vi "SSS_V3.1.vi"() -> ()   [LabVIEW 2017]
uses:
  <vilib>/DAQmx/write.llb/DAQmx Write (Analog 2D DBL NChan NSamp).vi
  <vilib>/DAQmx/read.llb/DAQmx Read (Analog 1D Wfm NChan NSamp).vi
  <vilib>/DAQmx/create/channels.llb/DAQmx Create Channel (AO-Voltage-Basic).vi
  <vilib>/DAQmx/configure/timing.llb/DAQmx Timing (Sample Clock).vi
  <vilib>/DAQmx/miscellaneous.llb/DAQmx Fill In Error Info.vi
  <vilib>/DAQmx/create/channels.llb/DAQmx Create Channel (AI-Voltage-Basic).vi
panel:
  out "Sampling Rate(EN, OSC)":dbl format="%#_3p"
  in  "TXEN_Pulse length(sec)":dbl=0.0004 format="%#_6p"
  in  "OSC_Pulse length(sec)":dbl=0.0004 format="%#_6p"
  in  "GAIN_Pulse length(sec)":dbl=1.0 format="%#_6p"
  in  "STC_Sampling Frequency(Hz)":dbl=192000.0 format="%0.2f"
  in  "STC_STEP":enum16{"0", "1", "2", "3", "4", "5", "6", "7"}(ring)
  in  "STC_Pulse length(sec)":dbl=1.0 format="%#_6p"
  in  "OSC_Frequency(Hz)":dbl=430000.0 format="%#_6p"
  in  "디바이스 이름(DAQ4)":tag="Dev4"
  in  "송신채널(DAQ4)":tag="Dev4/ao0:1"
  in  "송신채널(DAQ5)":tag="Dev5/ao0:1"
  in  "디바이스 이름(DAQ5)":tag="Dev5"
  in  "송신채널(DAQ3)":tag="Dev3/ao0:1"
  in  "Samplig Rate(RX)":dbl=1500000.0
  in  "RX time(sec)":dbl=0.0004
  out "RX.CH2 2":waveform(dbl)(graph)
  out "RX.CH2":waveform(dbl)(graph)
  in  "Start Frequency(Hz)":dbl=430000.0 format="%#_6p"
  in  "Pulse length(sec)":dbl=4e-06 format="%#_6p"
  in  "sampling rate(TX)":dbl=3760000.0 caption="Sampling Rate(TX)" format="%#.2g"
  in  "STEP":i32=100
  in  "초기 위상":dbl format="%#_13g"
  in  "Bandwidth":dbl=40000.0 format="%#_6p"
  out "Hz/1STEP":dbl
  out "TX.CH1":waveform(dbl)(graph)
  out "TX Spectrum":cluster{"f0":dbl, "df":dbl, "magnitude":dbl[]}(graph)
  out "TX.CH 2":waveform(dbl)(graph)
  in  "디바이스 이름(DAQ3)":tag="Dev3"
  in  "수신채널(DAQ3)":tag="Dev3/ai0:1"
  in  "Number of Sample":i32=150000 format="%#.0g"
  out "불리언 2":bool
  in  "Signal_Processing 2":bool
  out "CMD_PWD_DATA":i32=4
  in  "Signal_Processing":bool
  out "CMD_PWD":i32=7
  out "CMD_TVG":i32=6
  out "CMD_TVG_DATA":i32=4
  out "CMD_GAIN":i32=5
  out "CMD_GAIN_DATA":i32=255
  out "CMD_RANGE":i32=4
  out "CMD_RANGE_DATA":i32=100
  out "CMD_STOP":i32=3
  out "CMD_STOP_DATA":i32
  out "CMD_START":i32=2
  out "CMD_START_DATA":i32=1
  in  "port":u16=2500
  in  "address":string="30.0.1.18"
  in  "TCP/IP":bool
  in  "Server Closed":string="The server VI closed the connection."
  # "TCP/IP 소켓 통신 설정"
  # "송신 신호 변조 설정"
  # "수신 신호 변조 설정"
  # "DAQ Max 설정"
  # "DAQ3"
  # "DAQ5"
  # "DAQ4"
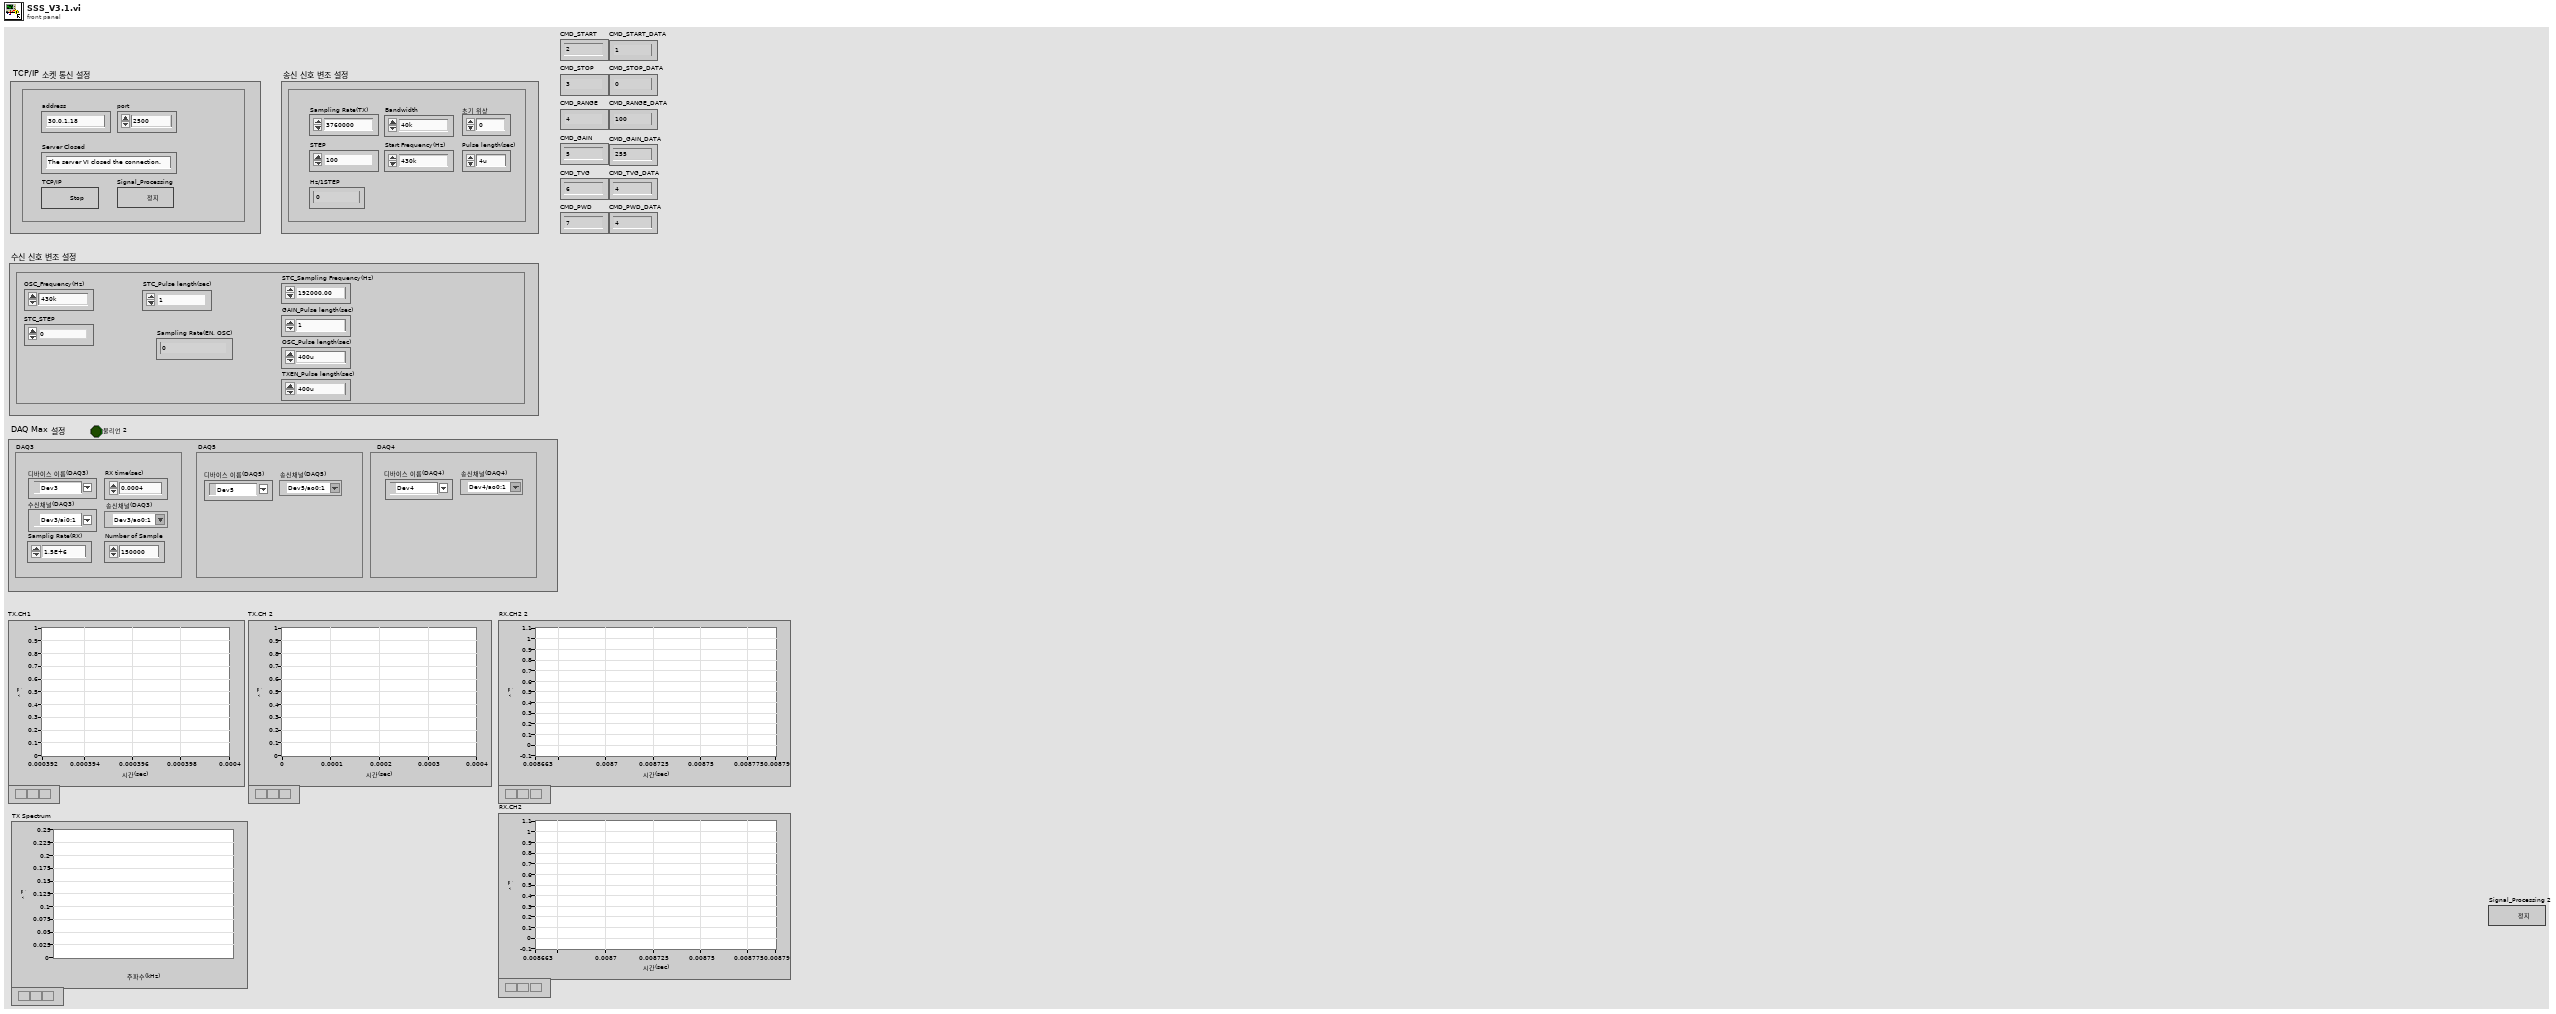
[diagram p1: front panel]
types:
  T1 = enum16{"Standard", "Buffered", "CRLF", "Immediate"}
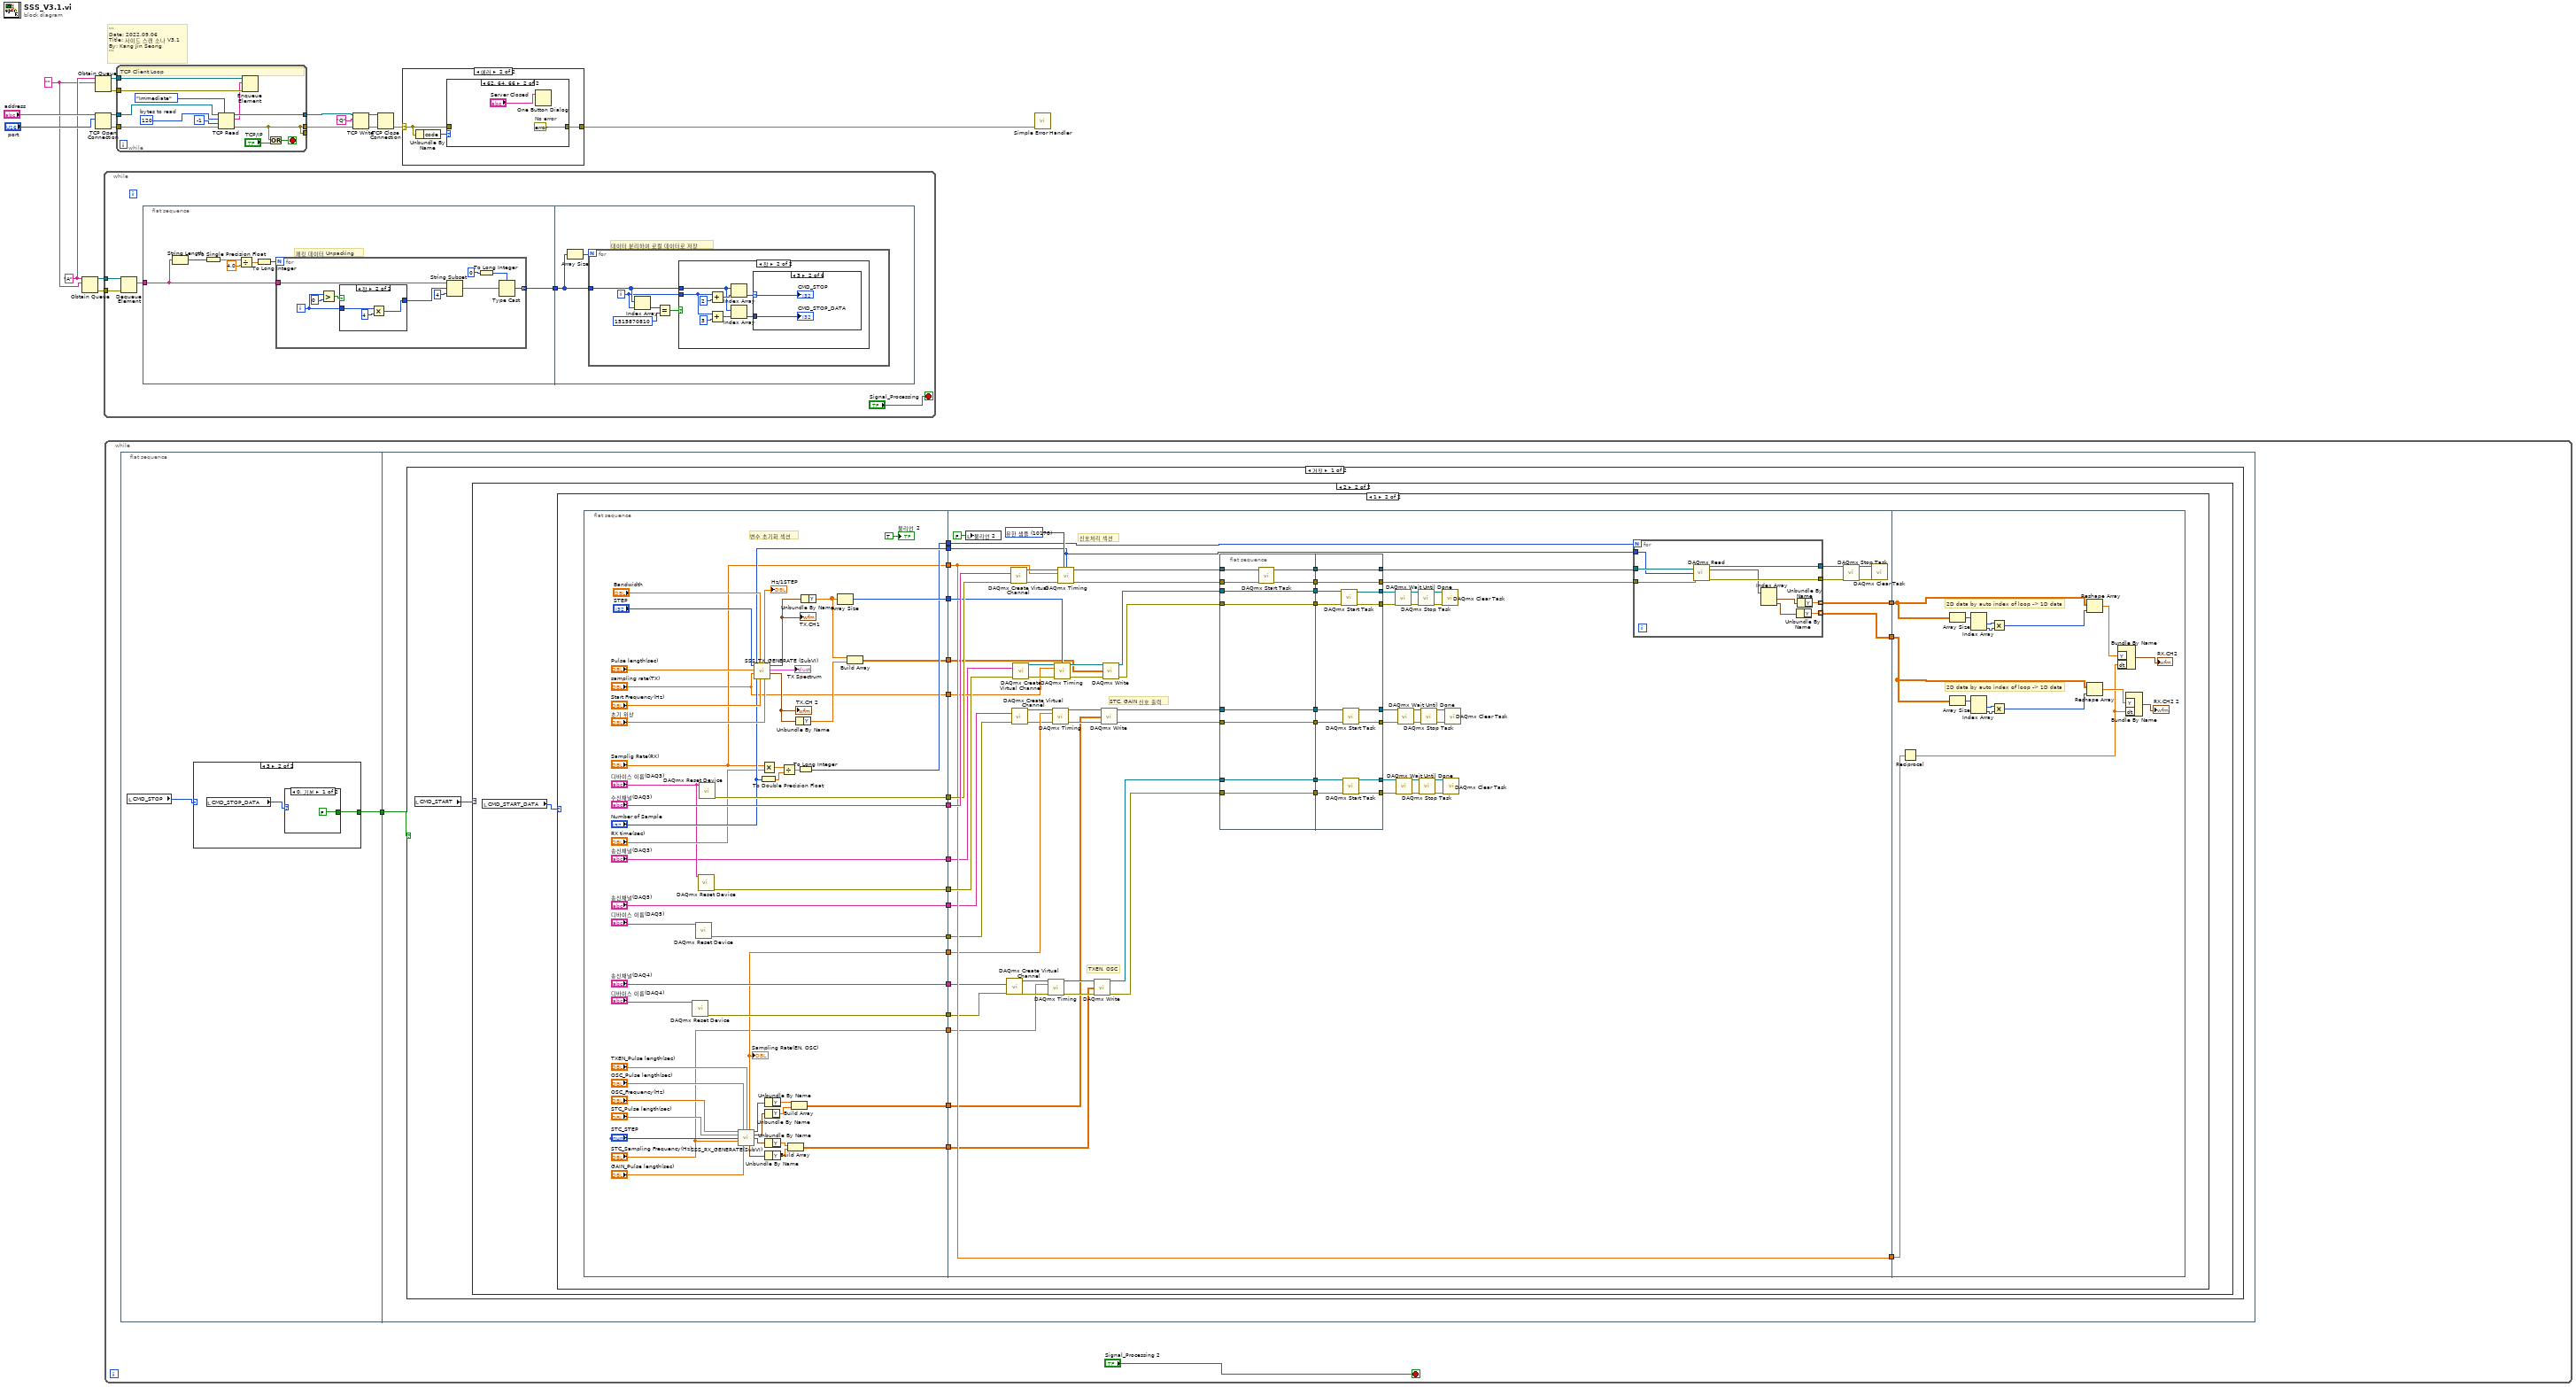
[diagram p0: block diagram]
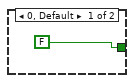
[diagram p2: hidden frame]
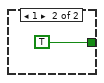
[diagram p3: hidden frame]
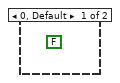
[diagram p4: hidden frame]
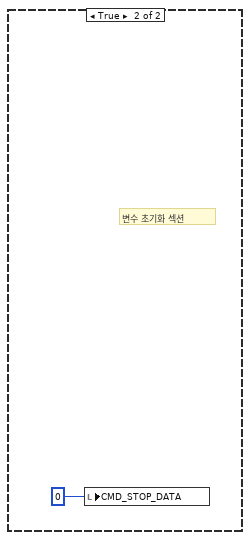
[diagram p6: hidden frame]
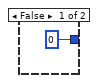
[diagram p7: hidden frame]
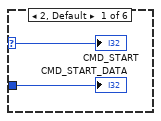
[diagram p9: hidden frame]
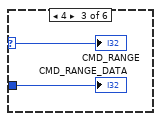
[diagram p10: hidden frame]
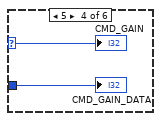
[diagram p11: hidden frame]
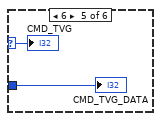
[diagram p12: hidden frame]
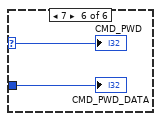
[diagram p13: hidden frame]
diagram:
  w1 = ""
  w4 = "A" ("이름(이름없음)")
  # "'''\nDate: 2022.09.06\nTitle: 사이드 스캔 소나 V3.1\nBy: Kang Jin Seong\n'''"
  n1 = Obtain Queue(name (unnamed)=w4, element data type=w1) -> (queue out=w3:refnum<queue>, error out=w2:errorcluster)  [unwired: 3 in, 1 out]
  n2 = Obtain Queue(name (unnamed)=w4, element data type=w1) -> (queue out=w6:refnum<queue>, error out=w5:errorcluster)  [unwired: 3 in, 1 out]
  n3 = TCP Open Connection(address="address", remote port or service name="port") -> (connection ID=w7:refnum<k5>, error out=w8:errorcluster)  [unwired: 3 in]
  n4 = while {
    tunnel: w3 -> [w21]
    tunnel: w2 -> [w20]
    stop <- "Signal_Processing" stop-if-true
    n5 = Dequeue Element(queue=w21, error in (no error)=w20) -> (element=w19:string)  [unwired: 1 in, 3 out]
    n6 = flat-sequence {
      tunnel: w19 -> [w25]
      tunnel: [w23] -> w22
      tunnel: w22 -> [w44]
      frame #0 {
        # "패킷 데이터 Unpacking"
        n7 = String Length(string=w25) -> (length=w29:i32)
        n8 = To Single Precision Float(number=w29) -> (single precision float=w28:sgl)
        n9 = Divide(x=w28, y=sgl 4.0) -> (x/y=w26:sgl)
        n10 = To Long Integer(number=w26) -> (32bit integer=w24:i32)
        n11 = for {
          N: w24 -> [_]
          tunnel: w25 -> [w39]
          tunnel: [w36] -> w23 mode=indexing
          i -> [w31]
          n12 = Greater?(x=w31, y=0) -> (0:w33:bool)
          n13 = case shown="참" w33 {
            tunnel: [0 w41] -> w32
            tunnel: w31 -> [_ w43]
            frame False {
            }
            frame True {
              n14 = Multiply(x=w43, y=4) -> (x*y=w41:i32)
            }
          }
          n15 = String Subset(string=w39, offset (0)=w32, length (rest)=4 ("길이(나머지)")) -> (substring=w30:string)
          n16 = To Long Integer(number=0 ("숫자")) -> (32bit integer=w38:i32)
          n17 = Type Cast(type=w38, x=w30) -> (*(type *) &x=w36:i32)
        }
      }
      frame #1 {
        # "데이터 분리하여 로컬 데이터로 저장"
        n18 = Array Size(array=w44) -> (size(s)=w45:i32)
        n19 = for {
          N: w45 -> [_]
          tunnel: w44 -> [w47]
          i -> [w46]
          n20 = Index Array(array=w47, index=w46) -> (element=w50:i32)
          n21 = Equal?(x=w50, y=1515870810) -> (x = y?=w48:bool)
          n22 = case shown="참" w48 {
            tunnel: w47 -> [_ w52]
            tunnel: w46 -> [_ w53]
            frame False {
            }
            frame True {
              n23 = Add(x=w53, y=2) -> (x+y=w57:i32)
              n24 = Add(x=w53, y=3) -> (x+y=w54:i32)
              n25 = Index Array(array=w52, index=w57) -> (element=w56:i32)
              n26 = Index Array(array=w52, index=w54) -> (element=w51:i32)
              n27 = case shown="3" w56 {
                selector: w56 -> [w60 w62 w64 w66 w68 w70]
                tunnel: w51 -> [w59 w61 w63 w65 w67 w69]
                frame 2, Default {
                  "CMD_START" <- w60
                  "CMD_START_DATA" <- w59
                }
                frame 3 {
                  "CMD_STOP" <- w62
                  "CMD_STOP_DATA" <- w61
                }
                frame 4 {
                  "CMD_RANGE" <- w64
                  "CMD_RANGE_DATA" <- w63
                }
                frame 5 {
                  "CMD_GAIN" <- w66
                  "CMD_GAIN_DATA" <- w65
                }
                frame 6 {
                  "CMD_TVG" <- w68
                  "CMD_TVG_DATA" <- w67
                }
                frame 7 {
                  "CMD_PWD" <- w70
                  "CMD_PWD_DATA" <- w69
                }
              }
            }
          }
        }
      }
    }
  }
  n28 = while {
    stop <- "Signal_Processing 2" stop-if-true
    n29 = flat-sequence {
      tunnel: [w73] -> w71
      tunnel: w71 -> [w80]
      frame #0 {
        n30 = local read "CMD_STOP"() -> (w74:i32)
        n31 = case shown="3" w74 {
          tunnel: [FALSE w76] -> w73
          frame 0, Default {
          }
          frame 3 {
            n32 = local read "CMD_STOP_DATA"() -> (w77:i32)
            n33 = case shown="0, 기본" w77 {
              tunnel: [FALSE TRUE] -> w76
              frame 0, Default {
              }
              frame 1 {
              }
            }
          }
        }
      }
      frame #1 {
        n34 = case shown="거짓" w80 {
          frame False {
            n35 = local read "CMD_START"() -> (w81:i32)
            n36 = case shown="2" w81 {
              frame 0, Default {
                (unwired) FALSE
              }
              frame 2 {
                n37 = local read "CMD_START_DATA"() -> (w82:i32)
                n38 = case shown="1" w82 {
                  frame 0, Default {
                  }
                  frame 1 {
                    n39 = flat-sequence {
                      tunnel: ["수신채널(DAQ3)"] -> w103
                      tunnel: [w142] -> w102
                      tunnel: ["Samplig Rate(RX)"] -> w101
                      tunnel: ["Number of Sample"] -> w100
                      tunnel: [w140] -> w99
                      tunnel: [w138] -> w98
                      tunnel: [w137] -> w97
                      tunnel: [w133] -> w93
                      tunnel: ["송신채널(DAQ3)"] -> w92
                      tunnel: [w128] -> w91
                      tunnel: ["송신채널(DAQ5)"] -> w90
                      tunnel: ["sampling rate(TX)"] -> w89
                      tunnel: [w110] -> w88
                      tunnel: ["송신채널(DAQ4)"] -> w87
                      tunnel: [w122] -> w86
                      tunnel: ["STC_Sampling Frequency(Hz)"] -> w85
                      tunnel: [w111] -> w84
                      tunnel: [w104] -> w83
                      tunnel: [w208] -> w96
                      tunnel: w103 -> [w206]
                      tunnel: w102 -> [w205]
                      tunnel: w101 -> [w200]
                      tunnel: w100 -> [w199]
                      tunnel: w99 -> [w203]
                      tunnel: w98 -> [w202]
                      tunnel: w97 -> [w201]
                      tunnel: [w200] -> w95
                      tunnel: [w197] -> w94
                      tunnel: w93 -> [w196]
                      tunnel: w92 -> [w195]
                      tunnel: w91 -> [w190]
                      tunnel: w90 -> [w189]
                      tunnel: w89 -> [w198]
                      tunnel: w88 -> [w188]
                      tunnel: w87 -> [w173]
                      tunnel: w86 -> [w172]
                      tunnel: w85 -> [w167]
                      tunnel: w84 -> [w156]
                      tunnel: w83 -> [w155]
                      tunnel: w96 -> [w274]
                      tunnel: w95 -> [w273]
                      tunnel: w94 -> [w268]
                      frame #0 {
                        # "변수 초기화 섹션"
                        n40 = call <vilib>:"DAQmx Reset Device.vi"("device in"="디바이스 이름(DAQ4)") -> ("error out"=w122:errorcluster)  [unwired: 1 in, 13 out]
                        n41 = call <vilib>:"DAQmx Reset Device.vi"("device in"="디바이스 이름(DAQ5)") -> ("error out"=w128:errorcluster)  [unwired: 1 in, 13 out]
                        n42 = call <vilib>:"DAQmx Reset Device.vi"("device in"="디바이스 이름(DAQ3)") -> ("error out"=w137:errorcluster)  [unwired: 1 in, 13 out]
                        n43 = call <vilib>:"DAQmx Reset Device.vi"("device in"="디바이스 이름(DAQ3)") -> ("error out"=w142:errorcluster)  [unwired: 1 in, 13 out]
                        n44 = call "SSS_RX_GENERATE(SubVI).vi"("OSC_Frequency(Hz)"="OSC_Frequency(Hz)", "OSC_Pulse length(sec)"="OSC_Pulse length(sec)", "TXEN_Pulse length(sec)"="TXEN_Pulse length(sec)", "STC_Pulse length(sec)"="STC_Pulse length(sec)", "STC_STEP"="STC_STEP", "STC_Sampling Frequency(Hz)"="STC_Sampling Frequency(Hz)", "GAIN_Pulse length(sec)"="GAIN_Pulse length(sec)") -> ("Sampling Rate(EN, OSC)"=w110:dbl, "TXEN"=w115:waveform(dbl), "OSC"=w114:waveform(dbl), "STC"=w108:waveform(dbl), "GAIN"=w107:waveform(dbl))  [unwired: 3 in, 1 out]
                        "Sampling Rate(EN, OSC)" <- w110
                        n45 = call "SSS_TX_GENERATE (SubVI).vi"("초기 위상"="초기 위상", "Start Frequency(Hz)"="Start Frequency(Hz)", "Bandwidth"="Bandwidth", "sampling rate"="sampling rate(TX)", "Pulse length(sec)"="Pulse length(sec)", "STEP"="STEP") -> ("TX.CH1 2"=w136:waveform(dbl), "TX Spectrum"=→"TX Spectrum":cluster{"f0":dbl, "df":dbl, "magnitude":dbl[]}, "TX.CH1"=w141:waveform(dbl), "Hz/1STEP"=→"Hz/1STEP":dbl)  [unwired: 2 in]
                        "TX.CH1" <- w141
                        "TX.CH 2" <- w136
                        n46 = To Double Precision Float(number="Number of Sample") -> (double precision float=w147:dbl)
                        n47 = Multiply(x="Samplig Rate(RX)", y="RX time(sec)") -> (x*y=w146:dbl)
                        n48 = Unbundle By Name(w114) -> ("Y"=w112:dbl[])
                        n49 = Unbundle By Name(w115) -> ("Y"=w113:dbl[])
                        n50 = Unbundle By Name(w108) -> ("Y"=w106:dbl[])
                        n51 = Unbundle By Name(w107) -> ("Y"=w105:dbl[])
                        n52 = Divide(x=w146, y=w147) -> (x/y=w148:dbl)
                        n53 = Build Array(w106, w105) -> (w104:dbl[][])
                        n54 = Build Array(w113, w112) -> (w111:dbl[][])
                        n55 = Unbundle By Name(w136) -> ("Y"=w134:dbl[])
                        n56 = To Long Integer(number=w148) -> (32bit integer=w138:i32)
                        n57 = Unbundle By Name(w141) -> ("Y"=w135:dbl[])
                        n58 = Array Size(array=w135) -> (size(s)=w140:i32)
                        n59 = Build Array(w135, w134) -> (w133:dbl[][])
                        "불리언 2" <- TRUE
                      }
                      frame #1 {
                        w204 = 10178 items=["유한 샘플"=10178, "연속 샘플"=10123, "하드웨어 타이밍에 의한 단일 포인트"=12522] ("sample mode")
                        # "TXEN, OSC"
                        # "STC, GAIN 신호 출력"
                        # "신호처리 섹션"
                        n60 = local write "불리언 2"(FALSE) -> ()
                        n61 = call-poly <vilib>:"DAQmx Create Virtual Channel.vi"("physical channels"=w173, "error in"=w172) -> ("task out"=w171:refnum<k21>, "error out"=w170:errorcluster)  [unwired: 7 in, 5 out]
                        n62 = call-poly <vilib>:"DAQmx Create Virtual Channel.vi"("physical channels"=w206, "error in"=w205) -> ("task out"=w227:refnum<k21>, "error out"=w228:errorcluster)  [unwired: 7 in, 5 out]
                        n63 = call-poly <vilib>:"DAQmx Create Virtual Channel.vi"("physical channels"=w189, "error in"=w190) -> ("task out"=w186:refnum<k21>, "error out"=w187:errorcluster)  [unwired: 7 in, 5 out]
                        n64 = call-poly <vilib>:"DAQmx Create Virtual Channel.vi"("physical channels"=w195, "error in"=w201) -> ("task out"=w218:refnum<k21>, "error out"=w217:errorcluster)  [unwired: 7 in, 5 out]
                        n65 = call-poly <vilib>:"DAQmx Timing.vi"("task/channels in"=w171, "rate"=w167, "error in"=w170) -> ("task out"=w168:refnum<k21>, "error out"=w169:errorcluster)  [unwired: 4 in, 7 out]
                        n66 = call-poly <vilib>:"DAQmx Timing.vi"("task/channels in"=w186, "rate"=w188, "error in"=w187) -> ("task out"=w184:refnum<k21>, "error out"=w185:errorcluster)  [unwired: 4 in, 7 out]
                        n67 = call-poly <vilib>:"DAQmx Timing.vi"("task/channels in"=w218, "samples per channel"=w203, "rate"=w198, "error in"=w217) -> ("task out"=w215:refnum<k21>, "error out"=w216:errorcluster)  [unwired: 3 in, 7 out]
                        n68 = call-poly <vilib>:"DAQmx Timing.vi"("task/channels in"=w227, "sample mode"=w204, "samples per channel"=w199, "rate"=w200, "error in"=w228) -> ("task out"=w226:refnum<k21>, "error out"=w225:errorcluster)  [unwired: 2 in, 7 out]
                        n69 = call-poly <vilib>:"DAQmx Write.vi"("task/channels in"=w168, "data"=w155, "error in"=w169) -> ("task out"=w164:refnum<k21>, "error out"=w163:errorcluster)  [unwired: 10 in, 1 out]
                        n70 = call-poly <vilib>:"DAQmx Write.vi"("task/channels in"=w184, "data"=w156, "error in"=w185) -> ("task out"=w182:refnum<k21>, "error out"=w180:errorcluster)  [unwired: 10 in, 1 out]
                        n71 = call-poly <vilib>:"DAQmx Write.vi"("task/channels in"=w215, "data"=w196, "error in"=w216) -> ("task out"=w194:refnum<k21>, "error out"=w191:errorcluster)  [unwired: 10 in, 1 out]
                        n72 = flat-sequence {
                          tunnel: [w250] -> w230
                          tunnel: [w249] -> w229
                          tunnel: w226 -> [w248]
                          tunnel: w225 -> [w247]
                          tunnel: w194 -> [w246]
                          tunnel: [w246] -> w193
                          tunnel: w191 -> [w245]
                          tunnel: [w245] -> w192
                          tunnel: w182 -> [w244]
                          tunnel: [w244] -> w183
                          tunnel: w180 -> [w243]
                          tunnel: [w243] -> w181
                          tunnel: w164 -> [w242]
                          tunnel: [w242] -> w166
                          tunnel: w163 -> [w241]
                          tunnel: [w241] -> w165
                          tunnel: w230 -> [w264]
                          tunnel: [w264] -> w223
                          tunnel: [w263] -> w224
                          tunnel: w229 -> [w263]
                          tunnel: [w262] -> w210
                          tunnel: [w261] -> w209
                          tunnel: w193 -> [w260]
                          tunnel: w192 -> [w259]
                          tunnel: w183 -> [w258]
                          tunnel: w181 -> [w257]
                          tunnel: [w256] -> w177
                          tunnel: [w255] -> w176
                          tunnel: w166 -> [w254]
                          tunnel: w165 -> [w253]
                          tunnel: [w252] -> w158
                          tunnel: [w251] -> w157
                          frame #0 {
                            n73 = call <vilib>:"DAQmx Start Task.vi"("task/channels in"=w248, "error in"=w247) -> ("task out"=w249:refnum<k21>, "error out"=w250:errorcluster)  [unwired: 12 in]
                          }
                          frame #1 {
                            n74 = call <vilib>:"DAQmx Start Task.vi"("task/channels in"=w260, "error in"=w259) -> ("task out"=w262:refnum<k21>, "error out"=w261:errorcluster)  [unwired: 12 in]
                            n75 = call <vilib>:"DAQmx Start Task.vi"("task/channels in"=w258, "error in"=w257) -> ("task out"=w256:refnum<k21>, "error out"=w255:errorcluster)  [unwired: 12 in]
                            n76 = call <vilib>:"DAQmx Start Task.vi"("task/channels in"=w254, "error in"=w253) -> ("task out"=w252:refnum<k21>, "error out"=w251:errorcluster)  [unwired: 12 in]
                          }
                        }
                        n77 = call <vilib>:"DAQmx Wait Until Done.vi"("task/channels in"=w210, "error in"=w209) -> ("task out"=w212:refnum<k21>, "error out"=w211:errorcluster)  [unwired: 12 in]
                        n78 = call <vilib>:"DAQmx Wait Until Done.vi"("task/channels in"=w158, "error in"=w157) -> ("task out"=w160:refnum<k21>, "error out"=w161:errorcluster)  [unwired: 12 in]
                        n79 = call <vilib>:"DAQmx Wait Until Done.vi"("task/channels in"=w177, "error in"=w176) -> ("task out"=w175:refnum<k21>, "error out"=w178:errorcluster)  [unwired: 12 in]
                        n80 = call <vilib>:"DAQmx Stop Task.vi"("task/channels in"=w212, "error in"=w211) -> ("task out"=w214:refnum<k21>, "error out"=w213:errorcluster)  [unwired: 12 in]
                        n81 = call <vilib>:"DAQmx Stop Task.vi"("task/channels in"=w160, "error in"=w161) -> ("task out"=w159:refnum<k21>, "error out"=w162:errorcluster)  [unwired: 12 in]
                        n82 = call <vilib>:"DAQmx Stop Task.vi"("task/channels in"=w175, "error in"=w178) -> ("task out"=w174:refnum<k21>, "error out"=w179:errorcluster)  [unwired: 12 in]
                        n83 = call <vilib>:"DAQmx Clear Task.vi"("task in"=w214, "error in"=w213) -> ()  [unwired: 13 in, 1 out]
                        n84 = call <vilib>:"DAQmx Clear Task.vi"("task in"=w159, "error in"=w162) -> ()  [unwired: 13 in, 1 out]
                        n85 = call <vilib>:"DAQmx Clear Task.vi"("task in"=w174, "error in"=w179) -> ()  [unwired: 13 in, 1 out]
                        n86 = for {
                          N: w202 -> [_]
                          tunnel: w224 -> [w240]
                          tunnel: w223 -> [w239]
                          tunnel: [w238] -> w222
                          tunnel: [w237] -> w219
                          tunnel: [w236] -> w208 mode=indexing
                          tunnel: w199 -> [w235]
                          tunnel: [w231] -> w197 mode=indexing
                          n87 = call-poly <vilib>:"DAQmx Read.vi"("task/channels in"=w240, "number of samples per channel"=w235, "error in"=w239) -> ("task out"=w237:refnum<k21>, "data"=w234:waveform(dbl)[], "error out"=w238:errorcluster)  [unwired: 10 out]
                          n88 = Index Array(array=w234) -> (element #1=w233:waveform(dbl), element #2=w232:waveform(dbl))  [unwired: 2 in]
                          n89 = Unbundle By Name(w232) -> ("Y"=w231:dbl[])
                          n90 = Unbundle By Name(w233) -> ("Y"=w236:dbl[])
                        }
                        n91 = call <vilib>:"DAQmx Stop Task.vi"("task/channels in"=w219, "error in"=w222) -> ("task out"=w220:refnum<k21>, "error out"=w221:errorcluster)  [unwired: 12 out]
                        n92 = call <vilib>:"DAQmx Clear Task.vi"("task in"=w220, "error in"=w221) -> ()  [unwired: 14 out]
                      }
                      frame #2 {
                        # "2D data by auto index of loop -> 1D data"
                        # "2D data by auto index of loop -> 1D data"
                        n93 = Reciprocal(x=w273) -> (1/x=w266:dbl)
                        n94 = Array Size(array=w274) -> (size(s)=w278:i32[])
                        n95 = Array Size(array=w268) -> (size(s)=w270:i32[])
                        n96 = Index Array(array=w278) -> (element #1=w279:i32, element #2=w275:i32)  [unwired: 2 in]
                        n97 = Index Array(array=w270) -> (element #1=w271:i32, element #2=w269:i32)  [unwired: 2 in]
                        n98 = Multiply(x=w279, y=w275) -> (x*y=w280:i32)
                        n99 = Multiply(x=w271, y=w269) -> (x*y=w272:i32)
                        n100 = Reshape Array(w274, w280) -> (w277:dbl[])
                        n101 = Reshape Array(w268, w272) -> (w267:dbl[])
                        n102 = Bundle By Name("Y"=w277, "dt"=w266) -> (→"RX.CH2":waveform(dbl))  [unwired: 1 in]
                        n103 = Bundle By Name("Y"=w267, "dt"=w266) -> (→"RX.CH2 2":waveform(dbl))  [unwired: 1 in]
                      }
                    }
                  }
                }
              }
            }
          }
          frame True {
            # "변수 초기화 섹션"
            n104 = local write "CMD_STOP_DATA"(0) -> ()
          }
        }
      }
    }
  }
  n105 = while {
    tunnel: [w291] -> w16
    tunnel: [w284] -> w14
    tunnel: w8 -> [w289]
    tunnel: w7 -> [w288]
    tunnel: w6 -> [w287]
    tunnel: w5 -> [w286]
    tunnel: [w284] -> _
    stop <- w292 stop-if-true
    w293 = 120  # bytes to read
    # "TCP Client Loop"
    n106 = TCP Read(connection ID=w288, bytes to read=w293, error in (no error)=w289, 7:T1."Immediate" ("모드(standard)"), 9:-1 ("타임아웃 ms (25000)")) -> (connection ID out=w291:refnum<k5>, data out=w282:string, error out=w284:errorcluster)
    n107 = Enqueue Element(queue=w287, element=w282, error in (no error)=w286) -> ()  [unwired: 1 in, 3 out]
    n108 = Or(x=w284, y="TCP/IP") -> (x .or. y?=w292:bool)
  }
  n109 = TCP Write(connection ID=w16, data in="Q", error in (no error)=w14) -> (connection ID out=w17:refnum<k5>, error out=w15:errorcluster)  [unwired: 2 out]
  n110 = TCP Close Connection(connection ID=w17, error in (no error)=w15) -> (error out=w12:errorcluster)  [unwired: 1 in, 1 out]
  n111 = case shown="에러" w12 {
    selector: w12 -> [w294 w296]
    tunnel: [w294 w295] -> w11
    frame No Error {
    }
    frame Error {
      n112 = Unbundle By Name(w296) -> ("code"=w297:i32)
      n113 = case shown="62, 64, 66" w297 {
        tunnel: w296 -> [w298 _]
        tunnel: [w298 w300] -> w295
        frame Default {
        }
        frame 62, 64, 66 {
          w300 = errorcluster {"status"=FALSE, "code"=0, "source"=""}  # No error
          n114 = One Button Dialog(message="Server Closed") -> ()  [unwired: 1 in, 1 out]
        }
      }
    }
  }
  n115 = call <vilib>:"Simple Error Handler.vi"("error in (no error)"=w11) -> ()  [unwired: 4 in, 5 out]
